vi "RGB to Depth.vi"(7 "RGB":u32) -> (8 "Depth Pixel":u8, 13 "Depth":dbl)   [LabVIEW 2018]
uses:
  <vilib>/vision/NI_Vision_Development_Module.lvlib
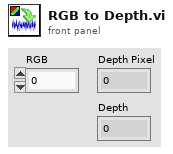
[diagram p1: front panel]
types:
  T1 = cluster{"Red (or Hue) value":u8, "Green (or Sat) value":u8, "Blue (or Light or Val) value":u8}
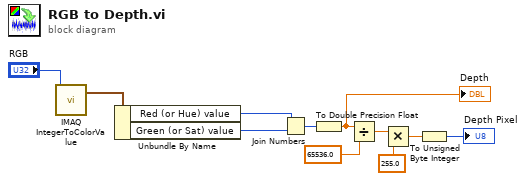
[diagram p0: block diagram]
diagram:
  n1 = call "IMAQ IntegerToColorValue"("U32 value"="RGB") -> ("Color Value"=w10:T1)  [unwired: 4 in, 3 out]
  n2 = Unbundle By Name(w10) -> ("Red (or Hue) value"=w9:u8, "Green (or Sat) value"=w8:u8)
  n3 = Join Numbers(hi=w9, lo=w8) -> ((hi.lo)=w7:u16)
  n4 = To Double Precision Float(number=w7) -> (double precision float=w6:dbl)
  "Depth" <- w6
  n5 = Divide(x=w6, y=65536.0) -> (x/y=w4:dbl)
  n6 = Multiply(x=w4, y=255.0) -> (x*y=w2:dbl)
  n7 = To Unsigned Byte Integer(number=w2) -> (unsigned 8bit integer=→"Depth Pixel":u8)
